vi "NetworkConfigExample.vi"() -> ()   [LabVIEW 2016]
doc: "This example VI demonstrates the use of Hyperion network sub-VIs for configuring static or dynamic (DHCP) network addresses on Hyperion instruments."
uses:
  <vilib>/Utility/miscctls.llb/LVPointTypeDef.ctl
  <vilib>/Utility/miscctls.llb/LVRectTypeDef.ctl
  h.Library/COMM/CTL/h.COMM.Socket Type.ctl
  h.Library/NET/CTL/h.NET.NetworkMode.ctl
  h.Library.lvlib
panel:
  in  "Stop Button":bool
  in  "ip address:":string="10.0.0.55"
  in  "Static IP Address":string
  in  "Static Netmask":string
  in  "Static Gateway":string
  in  "IP Address Mode":T1(radio)
  in  "Execute":bool
  out "Error":errorcluster
  # "hyperion network configuration example"
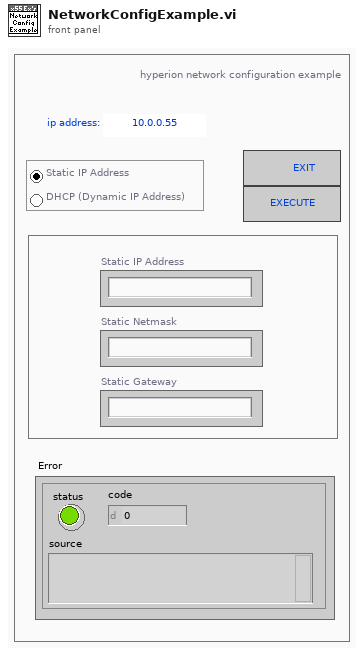
[diagram p1: front panel]
types:
  T1 = enum32{"Static IP Address", "DHCP (Dynamic IP Address)"}
  T2 = typedef "LVRectTypeDef.ctl" = cluster{"Left":i16, "Top":i16, "Right":i16, "Bottom":i16}
  T3 = typedef "LVPointTypeDef.ctl" = cluster{"Horizontal":i16, "Vertical":i16}
  T4 = enum8{"Enabled", "Disabled", "Disabled and Grayed Out"}
  T5 = typedef "h.Library.lvlib/h.NET.NetworkMode.ctl" = enum8{"Static", "DHCP"}
  T6 = typedef "h.Library.lvlib/h.COMM.Socket Type.ctl" = u16
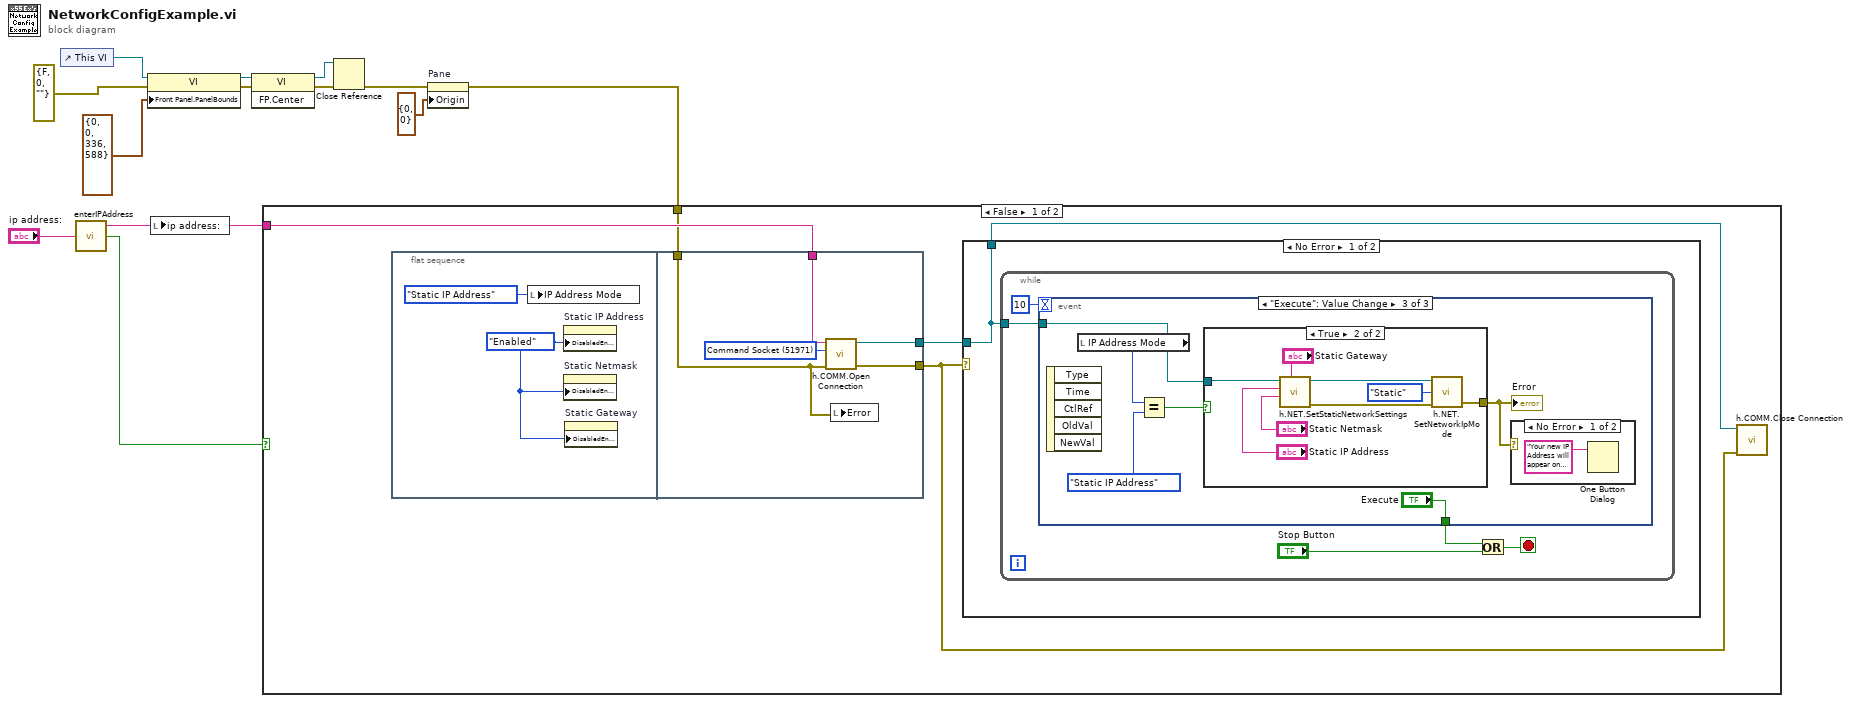
[diagram p0: block diagram]
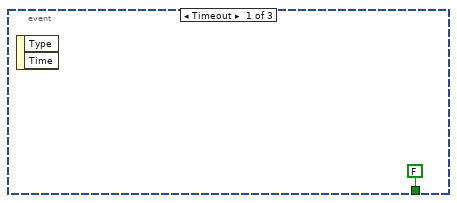
[diagram p2: hidden frame]
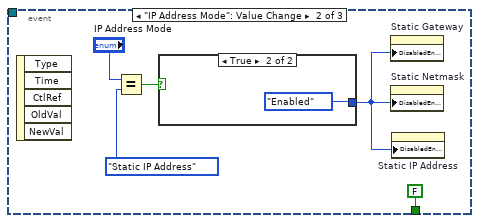
[diagram p3: hidden frame]
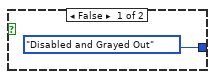
[diagram p4: hidden frame]
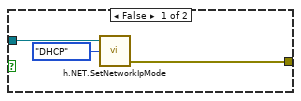
[diagram p6: hidden frame]
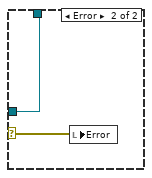
[diagram p7: hidden frame]
diagram:
  n1 = control-ref of="This VI"() -> (w2:refnum<vi>)
  n2 = call "enterIPAddress.vi"("IP Address"="ip address:") -> ("IP Address Out"=w11:string, "Was Canceled"=w12:bool)  [unwired: 1 in]
  n3 = property class="VI"(reference=w2, error in=errorcluster {"status"=FALSE, "code"=0, "source"=""}, "Front Panel.PanelBounds"=T2 {"Left"=0, "Top"=0, "Right"=336, "Bottom"=588} ("Front Panel Window:Panel Bounds 2")) -> (reference out=w3:refnum<vi>, error out=w5:errorcluster)
  n4 = local write "ip address:"(w11) -> ()
  n5 = invoke class="VI" method="FP.Center"(reference=w3, error in=w5) -> (reference out=w7:refnum<vi>, error out=w8:errorcluster)  [unwired: 1 in, 1 out]
  n6 = Close Reference(reference=w7, error in (no error)=w8) -> (error out=w9:errorcluster)
  n7 = property on="Pane" class="Pane"(error in=w9, "Origin"=T3 {"Horizontal"=0, "Vertical"=0}) -> (error out=w1:errorcluster)  [unwired: 1 in, 1 out]
  n8 = case shown="False" w12 {
    tunnel: w11 -> [w15 _]
    tunnel: w1 -> [w14 _]
    frame False {
      n9 = flat-sequence {
        tunnel: [w25] -> w18
        tunnel: [w24] -> w17
        tunnel: w15 -> [w22]
        tunnel: w14 -> [w21]
        frame #0 {
          w20 = T4."Enabled" ("Disabled")
          n10 = local write "IP Address Mode"(T1."Static IP Address" ("IP Address Mode")) -> ()
          n11 = property on="Static IP Address" class="Str"("DisabledEnum"=w20) -> ()  [unwired: 2 in, 2 out]
          n12 = property on="Static Netmask" class="Str"("DisabledEnum"=w20) -> ()  [unwired: 2 in, 2 out]
          n13 = property on="Static Gateway" class="Str"("DisabledEnum"=w20) -> ()  [unwired: 2 in, 2 out]
        }
        frame #1 {
          w23 = T6 51971 items=["Command Socket"=51971, "Streaming Data Socket"=51972] ("Port")
          n14 = call "h.COMM.Open Connection.vi"("error in"=w21, "Port"=w23, "Address"=w22) -> ("error out"=w25:errorcluster, "Connection ID"=w24:refnum<k5>)  [unwired: 7 in]
          n15 = local write "Error"(w21) -> ()
        }
      }
      n16 = case shown="No Error" w18 {
        selector: w18 -> [_ w58]
        tunnel: w17 -> [w26 w59]
        tunnel: [w26 w59] -> w16
        frame No Error {
          n17 = while {
            tunnel: w26 -> [w30]
            stop <- w31 stop-if-true
            n18 = event shown="[2] \"Execute\": Value Change" {
              selector: _ -> [_ _ _]
              dyn-events: _ -> [_ _ _]
              timeout: 10 -> [_ _ _]
              tunnel: w30 -> [_ _ w42]
              tunnel: [FALSE ("Execute") FALSE ("Execute") "Execute"] -> w27
              event Timeout {
                n19 = event-data() -> ()  [unwired: 1 in, 2 out]
              }
              event "IP Address Mode": Value Change {
                n20 = event-data() -> ()  [unwired: 1 in, 5 out]
                n21 = Equal?(x="IP Address Mode", y=T1."Static IP Address" ("IP Address Mode")) -> (x = y?=w35:bool)
                n22 = case shown="True" w35 {
                  tunnel: [T4."Disabled and Grayed Out" ("Disabled") T4."Enabled" ("Disabled")] -> w34
                  frame False {
                  }
                  frame True {
                  }
                }
                n23 = property on="Static Gateway" class="Str"("DisabledEnum"=w34) -> ()  [unwired: 2 in, 2 out]
                n24 = property on="Static Netmask" class="Str"("DisabledEnum"=w34) -> ()  [unwired: 2 in, 2 out]
                n25 = property on="Static IP Address" class="Str"("DisabledEnum"=w34) -> ()  [unwired: 2 in, 2 out]
              }
              event "Execute": Value Change {
                n26 = event-data() -> ()  [unwired: 1 in, 5 out]
                n27 = local read "IP Address Mode"() -> (w43:T1)
                n28 = Equal?(x=w43, y=T1."Static IP Address" ("IP Address Mode")) -> (x = y?=w45:bool)
                n29 = case shown="True" w45 {
                  tunnel: w42 -> [w48 w56]
                  tunnel: [w47 w50] -> w41
                  frame False {
                    n30 = call "h.NET.SetNetworkIpMode.vi"("Network Mode"=h.NET.NetworkMode."DHCP", "Connection ID"=w48) -> ("error out"=w47:errorcluster)  [unwired: 1 in, 2 out]
                  }
                  frame True {
                    n31 = call "h.NET.SetStaticNetworkSettings.vi"("Gateway"="Static Gateway", "Netmask"="Static Netmask", "IP Address"="Static IP Address", "Connection ID"=w56) -> ("error out"=w55:errorcluster, "Connection ID"=w54:refnum<k5>)  [unwired: 2 in, 1 out]
                    n32 = call "h.NET.SetNetworkIpMode.vi"("error in"=w55, "Network Mode"=h.NET.NetworkMode."Static", "Connection ID"=w54) -> ("error out"=w50:errorcluster)  [unwired: 2 out]
                  }
                }
                "Error" <- w41
                n33 = case shown="No Error" w41 {
                  frame No Error {
                    n34 = One Button Dialog(message="Your new IP Address will appear on the front of your unit momentarily.") -> ()  [unwired: 1 in, 1 out]
                  }
                  frame Error {
                  }
                }
              }
            }
            n35 = Or(x=w27, y="Stop Button") -> (x .or. y?=w31:bool)
          }
        }
        frame Error {
          n36 = local write "Error"(w58) -> ()
        }
      }
      n37 = call "h.COMM.Close Connection.vi"("error in"=w18, "Connection ID"=w16) -> ()  [unwired: 9 in, 1 out]
    }
    frame True {
    }
  }
